vi "1 Container Position 3.vi"(11 "Move Away Time":dbl=5.0 caption="Time Target (s)") -> ()   [LabVIEW 2014]
uses:
  1 Container States.ctl
  Robot Global Data.vi
  Desired Arm Position.vi
  <vilib>/Rock Robotics/WPI/RobotDrive/WPI_RobotDriveGetSetRefNum.vi
  <vilib>/Rock Robotics/WPI/RobotDrive/WPI_RobotDriveArcadeDrive_Standard(NoSaturation).vi
panel:
  out "Enum":T1=enum."Move Away"
  in  "Time Moving Forward":dbl=4.0
  in  "Speed":dbl=0.55
  in  "Desired Lift Height":dbl=5.0
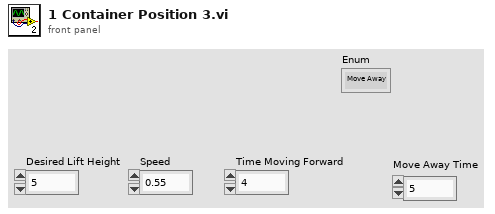
[diagram p1: front panel]
types:
  T1 = typedef "1 Container States.ctl" = enum16{"Start", "Grab Container", "Lift Container", "Move Forward", "Turn 90 Degrees", "Reset Gyro", "Move Away", "Stop"}
  T2 = typedef "WPI_RobotDriveDevRef.ctl" = cluster{"DevStatus":errorcluster, "Motors[]":T3[], "Square Inputs":bool, "Max Output":dbl}
  T3 = typedef "WPI_MotorControlDeviceRef.ctl" = cluster{"DeviceStatus":errorcluster, "Type":T4, "PWM":cluster{"Controller":T5, "PWM Channel":T6, "DeadBand":T7}, "CAN":cluster{"Device Number":u8, "Control Mode":T8, "Semaphore":T9, "Max Vout":dbl, "TalonSRX Control Mode":T10}, "Invert":bool, "TransformRef":T11, "InvTransformRef":T11}
  T4 = typedef "WPI_MotorControlType.ctl" = enum16{"PWM", "CAN", "CANTalonSRX"}
  T5 = typedef "FPGA_TypedefDigitalModule.ctl" = enum16{"Controller 1"}
  T6 = typedef "FPGA_DIOPWMChannel.ctl" = enum8{"PWM 0", "PWM 1", "PWM 2", "PWM 3", "PWM 4", "PWM 5", "PWM 6", "PWM 7", "PWM 8", "PWM 9", "PWM MXP 0", "PWM MXP 1", "PWM MXP 2", "PWM MXP 3", "PWM MXP 4", "PWM MXP 5", "PWM MXP 6", "PWM MXP 7", "PWM MXP 8", "PWM MXP 9", "Invalid"}
  T7 = typedef "WPI_PWMDeadband.ctl" = cluster{"Name":string, "maxPositivePwm":i32, "minPositivePwm":i32, "centerPwm":i32, "maxNegativePwm":i32, "minNegativePwm":i32, "angularRange":u16}
  T8 = typedef "WPI_CANJaguar_ControlMode.ctl" = enum8{"Percent VBus", "Current", "Speed", "Position", "Voltage"}
  T9 = typedef "Semaphore RefNum" = refnum<k1>
  T10 = typedef "WPI_CANTalonSRX_APIControlMode.ctl" = enum8{"Percent VBus", "Speed", "Position", "Slave", "Unchanged / Invalid"}
  T11 = typedef "WPI_PWMTransform_ConPane.ctl" = refnum<vi>
  T12 = typedef "WPI_GyroDevRef.ctl" = cluster{"DevStatus":errorcluster, "Analog Module":T13, "Analog Channel":T14, "Offset":dbl, "Gain (VoltsPerDegree/Second)":dbl}
  T13 = typedef "FPGA_TypedefAnalogModule.ctl" = enum16{"Controller 1"}
  T14 = typedef "FPGA_AIChannel.ctl" = enum8{"AI 0", "AI 1", "AI 2", "AI 3", "AI MXP 0", "AI MXP 1", "AI MXP 2", "AI MXP 3", "Invalid"}
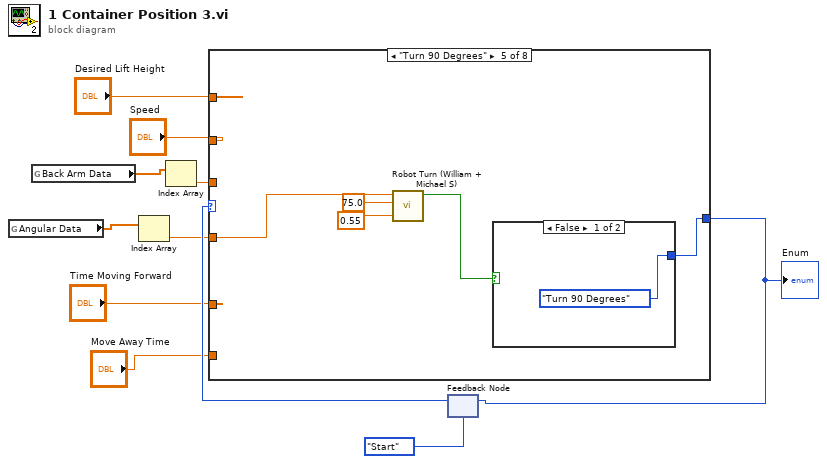
[diagram p0: block diagram]
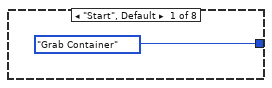
[diagram p2: hidden frame]
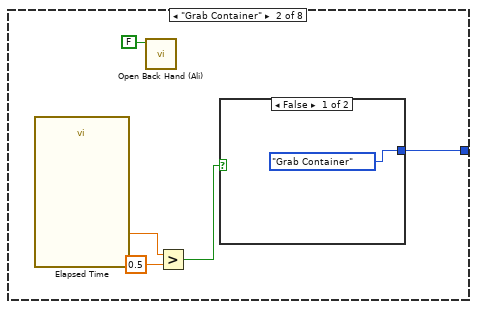
[diagram p3: hidden frame]
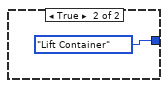
[diagram p4: hidden frame]
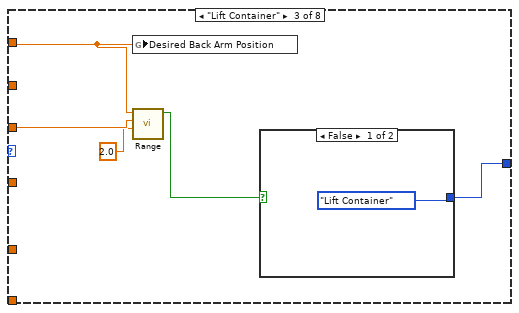
[diagram p5: hidden frame]
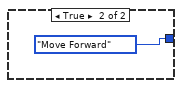
[diagram p6: hidden frame]
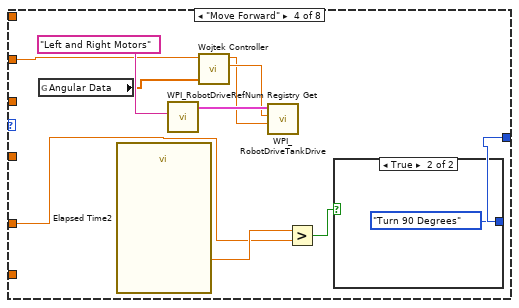
[diagram p7: hidden frame]
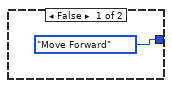
[diagram p8: hidden frame]
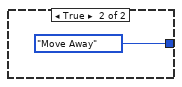
[diagram p9: hidden frame]
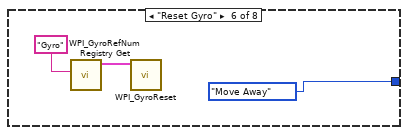
[diagram p10: hidden frame]
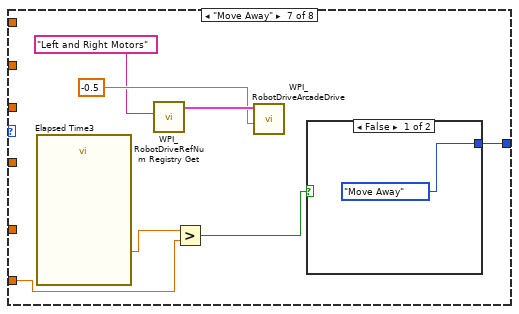
[diagram p11: hidden frame]
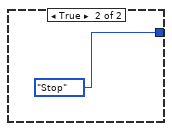
[diagram p12: hidden frame]
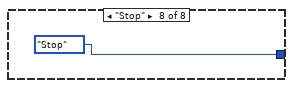
[diagram p13: hidden frame]
diagram:
  n1 = global read "Robot Global Data.vi" "Angular Data"() -> (w3:dbl[])
  n2 = global read "Robot Global Data.vi" "Back Arm Data"() -> (w7:dbl[])
  n3 = Index Array(array=w3) -> (element=w2:dbl)  [unwired: 1 in]
  n4 = Index Array(array=w7) -> (element=w6:dbl)  [unwired: 1 in]
  n5 = feedback #1(1_Container_States."Start") -> (w10:T1)
  n6 = case shown="\"Turn 90 Degrees\"" w10 {
    tunnel: [1_Container_States."Grab Container" w17 w20 w32 w40 1_Container_States."Move Away" w55 1_Container_States."Stop"] -> w9
    tunnel: "Desired Lift Height" -> [_ _ w23 _ _ _ _ _]
    tunnel: w6 -> [_ _ w24 _ _ _ _ _]
    tunnel: "Speed" -> [_ _ _ w29 _ _ _ _]
    tunnel: "Time Moving Forward" -> [_ _ _ w31 _ _ _ _]
    tunnel: w2 -> [_ _ _ _ w43 _ _ _]
    tunnel: "Move Away Time" -> [_ _ _ _ _ _ w51 _]
    frame "Start", Default {
    }
    frame "Grab Container" {
      n7 = call "Elapsed Time"() -> ("Elapsed Time (s)"=w16:dbl)  [unwired: 12 in, 7 out]
      n8 = call "Open Back Hand (Ali).vi"("Open?"=FALSE) -> ()  [unwired: 11 in]
      n9 = Greater?(x=w16, y=0.5) -> (0:w14:bool)
      n10 = case shown="False" w14 {
        tunnel: [1_Container_States."Grab Container" 1_Container_States."Lift Container"] -> w17
        frame False {
        }
        frame True {
        }
      }
    }
    frame "Lift Container" {
      n11 = global write "Desired Arm Position.vi" "Desired Back Arm Position"(w23) -> ()
      n12 = call "Range.vi"("Range"=2.0, "Input"=w24, "In Range of"=w23) -> ("In Range?"=w21:bool)  [unwired: 8 in]
      n13 = case shown="False" w21 {
        tunnel: [1_Container_States."Lift Container" 1_Container_States."Move Forward"] -> w20
        frame False {
        }
        frame True {
        }
      }
    }
    frame "Move Forward" {
      n14 = global read "Robot Global Data.vi" "Angular Data"() -> (w30:dbl[])
      n15 = call "Elapsed Time2"() -> ("Elapsed Time (s)"=w34:dbl)  [unwired: 12 in, 7 out]
      n16 = call <vilib>:"WPI_RobotDriveRefNum Registry Get.vi"("refnum name"="Left and Right Motors") -> ("RobotDriveDevRef"=w36:T2)  [unwired: 9 in, 1 out]
      n17 = call "Wojtek Controller.vi"("Current Angle"=w30, "Speed"=w29) -> ("left axis value"=w28:dbl, "right axis value"=w27:dbl)  [unwired: 8 in]
      n18 = call <vilib>:"WPI_RobotDriveTankDrive.vi"("Right axis value"=w27, "Left axis value"=w28, "RobotDriveDevRef"=w36) -> ()  [unwired: 6 in, 3 out]
      n19 = Greater?(x=w34, y=w31) -> (0:w33:bool)
      n20 = case shown="True" w33 {
        tunnel: [1_Container_States."Move Forward" 1_Container_States."Turn 90 Degrees"] -> w32
        frame False {
        }
        frame True {
        }
      }
    }
    frame "Turn 90 Degrees" {
      n21 = call "Robot Turn (William + Michael S).vi"("X axis value"=0.55, "Desired Degree"=75.0, "Gyro Degrees"=w43) -> ("Stop"=w39:bool)  [unwired: 8 in]
      n22 = case shown="False" w39 {
        tunnel: [1_Container_States."Turn 90 Degrees" 1_Container_States."Move Away"] -> w40
        frame False {
        }
        frame True {
        }
      }
    }
    frame "Reset Gyro" {
      n23 = call <vilib>:"WPI_GyroRefNum Registry Get.vi"("refnum name"="Gyro") -> ("GyroDevRef"=w48:T12)  [unwired: 9 in, 1 out]
      n24 = call <vilib>:"WPI_GyroReset.vi"("GyroDevRef"=w48) -> ()  [unwired: 9 in, 2 out]
    }
    frame "Move Away" {
      n25 = call "Elapsed Time3"() -> ("Elapsed Time (s)"=w50:dbl)  [unwired: 12 in, 7 out]
      n26 = call <vilib>:"WPI_RobotDriveRefNum Registry Get.vi"("refnum name"="Left and Right Motors") -> ("RobotDriveDevRef"=w54:T2)  [unwired: 9 in, 1 out]
      n27 = Greater?(x=w50, y=w51) -> (0:w49:bool)
      n28 = call-poly <vilib>:"WPI_RobotDriveArcadeDrive.vi"("Y axis value"=-0.5 ("Speed"), "RobotDriveDevRef"=w54) -> ()  [unwired: 7 in, 3 out]
      n29 = case shown="False" w49 {
        tunnel: [1_Container_States."Move Away" 1_Container_States."Stop"] -> w55
        frame False {
        }
        frame True {
        }
      }
    }
    frame "Stop" {
    }
  }
  "Enum" <- w9
  n30 = feedback-in #1(w9) -> ()
